vi "I2C Write.vi"(5 "buffer":string, 6 "options":u32=6 format="%02x", 8 "error in (no error)":errorcluster, 11 "handle":u32 format="%08x") -> (0 "error out":errorcluster, 2 "sizeTransfered":u32, 3 "handle out":u32 format="%08x")   [LabVIEW 2024, in "libMPSSE-I2C.lvlib"]
doc: "FTDI_API FT_STATUS SPI_Write(FT_HANDLE handle, uint8 *buffer,\n uint32 sizeToTransfer, uint32 *sizeTransfered, uint32 options);"
uses:
  libMPSSE-I2C.lvlib
  libmpsse.dll
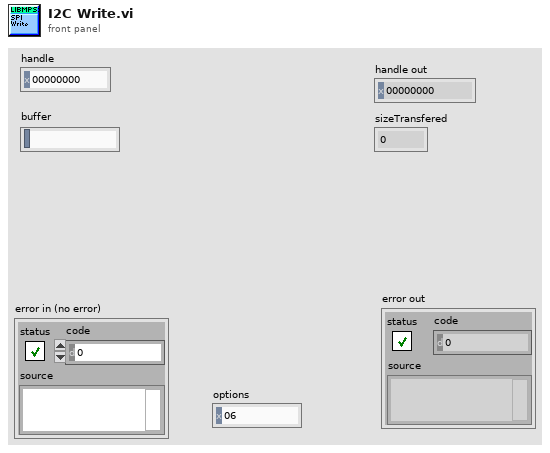
[diagram p1: front panel]
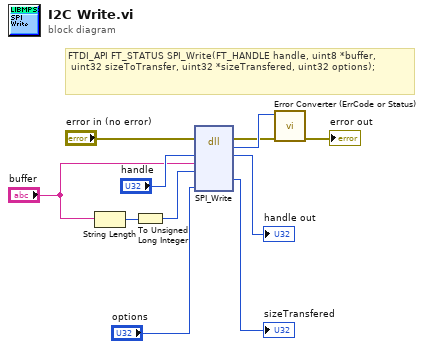
[diagram p0: block diagram]
diagram:
  # "FTDI_API FT_STATUS SPI_Write(FT_HANDLE handle, uint8 *buffer,\n\tuint32 sizeToTransfer, uint32 *sizeTransfered, uint32 options);"
  n1 = String Length(string="buffer") -> (length=w1:i32)
  n2 = To Unsigned Long Integer(number=w1) -> (unsigned 32bit integer=w2:u32)
  n3 = dll-call lib="C:/Workspace/sm_6576_001_RIB_Sequencer/I2C/libMPSSE.*" fn="SPI_Write"(error in="error in (no error)", "handle"="handle", "buffer"="buffer", "sizeToTransfer"=w2, "options"="options") -> (error out=w5:errorcluster, w11:u32, "handle"=→"handle out":u32, "sizeTransfered"=→"sizeTransfered":u32)  [unwired: 6 in, 1 out]
  n4 = call "Error Converter (ErrCode or Status).vi"("error in (no error)"=w5, "error code"=w11) -> ("error out"=→"error out":errorcluster)  [unwired: 9 in]
